vi "SetControlData.vi"(0 "reference in":refnum<class "WebFrontPanel.lvclass">, 1 "UID":i32, 2 "Value":string, 5 "error in (no error)":errorcluster) -> (14 "reference out":refnum<class "WebFrontPanel.lvclass">, 19 "error out":errorcluster)   [LabVIEW 2014, in "WebFrontPanel.lvclass"]
uses:
  WebFrontPanel.lvclass
  Object_class/Object.lvclass
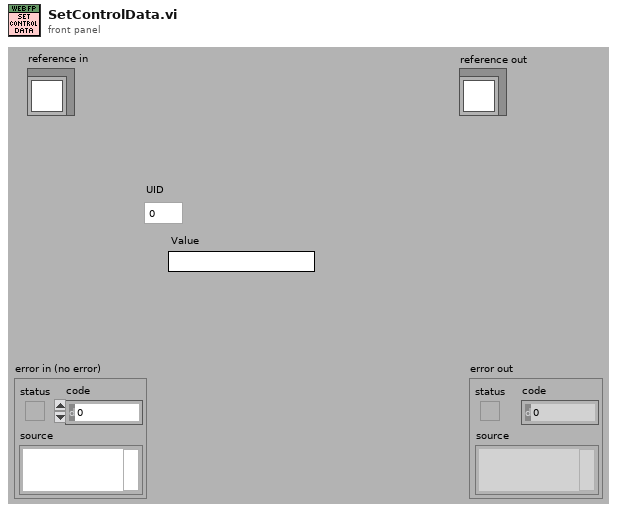
[diagram p1: front panel]
types:
  T1 = typedef "WebFrontPanel.lvclass/ObjectAttributes.ctl" = cluster{"VI Name":string, "VI Reference":refnum<vi>, "Queue To VI ":refnum<queue>, "Controls":refnum<class "Object.lvclass">[], "Indicators":refnum<class "Object.lvclass">[], "Decorations":refnum<class "Object.lvclass">[]}
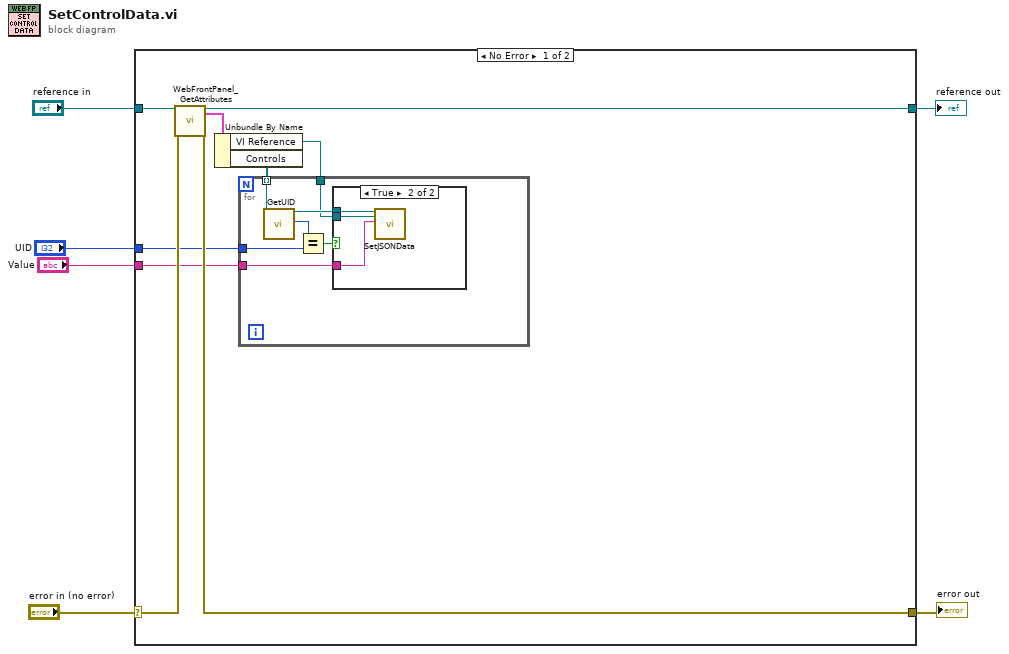
[diagram p0: block diagram]
diagram:
  n1 = case shown="No Error" "error in (no error)" {
    selector: "error in (no error)" -> [w15 w27]
    tunnel: [w13 w27] -> w5
    tunnel: [w11 w26] -> w3
    tunnel: "reference in" -> [w12 w26]
    tunnel: "UID" -> [w9 _]
    tunnel: "Value" -> [w7 _]
    frame No Error {
      n2 = call "WebFrontPanel_GetAttributes.vi"("reference in"=w12, "error in (no error)"=w15) -> ("reference out"=w11:refnum<class "WebFrontPanel.lvclass">, "Data"=w14:T1, "error out"=w13:errorcluster)  [unwired: 14 in, 1 out]
      n3 = Unbundle By Name(w14) -> ("VI Reference"=w8:refnum<vi>, "Controls"=w10:refnum<class "Object.lvclass">[])
      n4 = for {
        tunnel: w10 -> [w22] mode=indexing
        tunnel: w9 -> [w20]
        tunnel: w8 -> [w17]
        tunnel: w7 -> [w16]
        n5 = call-dynamic "GetUID.vi"("reference in"=w22) -> ("reference out"=w18:refnum<class "Object.lvclass">, "UID"=w21:i32)  [unwired: 16 in, 1 out]
        n6 = Equal?(x=w21, y=w20) -> (x = y?=w19:bool)
        n7 = case shown="True" w19 {
          tunnel: w18 -> [_ w25]
          tunnel: w17 -> [_ w24]
          tunnel: w16 -> [_ w23]
          frame False {
          }
          frame True {
            n8 = call-dynamic "SetJSONData.vi"("reference in"=w25, "VI Reference"=w24, "Value"=w23) -> ()  [unwired: 15 in, 2 out]
          }
        }
      }
    }
    frame Error {
    }
  }
  "error out" <- w5
  "reference out" <- w3
